vi "_Destroy.vi"(8 "error in (no error)":errorcluster, 11 "ClashRoyale in":refnum<class "StashRoyale.lvclass">) -> (0 "error out":errorcluster)   [LabVIEW 2020, in "StashRoyale.lvclass"]
uses:
  StashRoyale.lvclass
  StashRoyale.lvclass/StashRoyale.ctl
  <vilib>/drjdpowell/SQLite Library/SQL Connection/Connection.lvclass
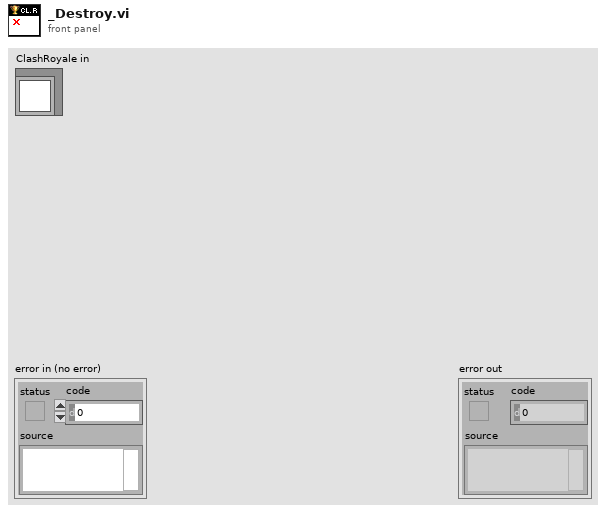
[diagram p1: front panel]
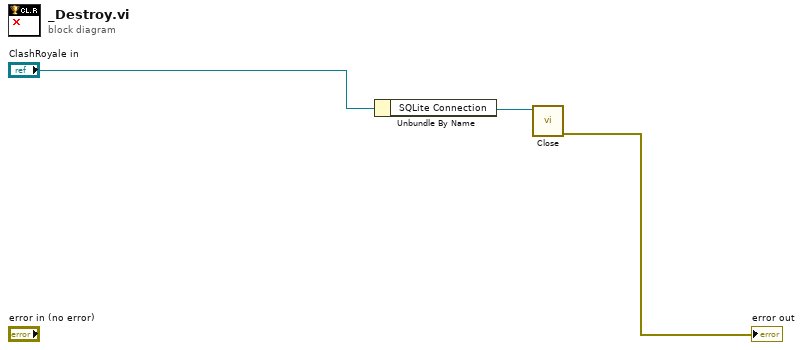
[diagram p0: block diagram]
diagram:
  n1 = Unbundle By Name("ClashRoyale in") -> ("SQLite Connection"=w1:refnum<class "Connection.lvclass">)
  n2 = call-dynamic "Close.vi"("SQLite Connection in"=w1) -> ("error out"=→"error out":errorcluster)  [unwired: 10 in]
